vi "execution class name.vi"(8 "error in":errorcluster, 11 "configuration in":refnum<class "CVT configuration.lvclass">) -> (0 "error out":errorcluster, 2 "execution class":string, 3 "configuration out":refnum<class "CVT configuration.lvclass">)   [LabVIEW 2013, in "CVT configuration.lvclass"]
uses:
  CVT configuration.lvclass
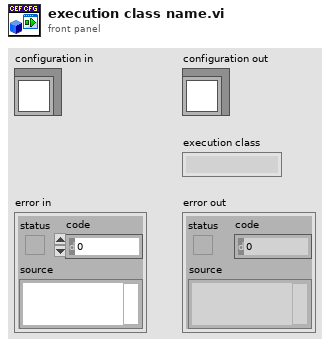
[diagram p1: front panel]
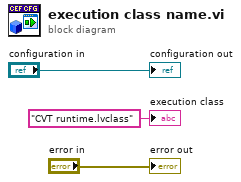
[diagram p0: block diagram]
diagram:
  "error out" <- "error in"
  "configuration out" <- "configuration in"
  "execution class" <- "CVT runtime.lvclass" ("execution class")
